vi "Subtract DAQ Offset.vi"(8 "error in (no error)":errorcluster, 11 "Instrument.DAQ":refnum<class "Instrument.DAQ.lvclass">) -> (0 "error out":errorcluster, 3 "Instrument.DAQ out":refnum<class "Instrument.DAQ.lvclass">)   [LabVIEW 2019, in "Instrument.Lockin.lvlib" / "Instrument.DAQ.lvclass"]
uses:
  Instrument.DAQ.lvclass
  Instrument.DAQ.lvclass/Instrument.DAQ.ctl
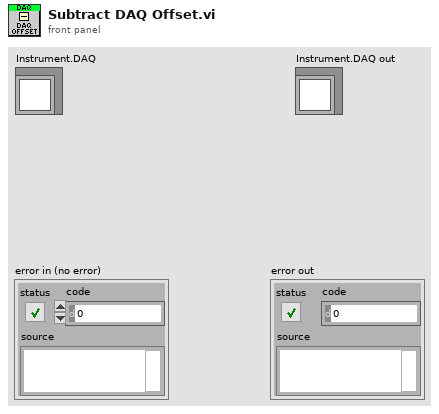
[diagram p1: front panel]
types:
  T1 = typedef "Instrument.Lockin.lvlib/Instrument.DAQ.lvclass/Channel.Gain--Cluster--Array.ctl" = T2[]
  T2 = typedef "Instrument.Lockin.lvlib/Instrument.DAQ.lvclass/Channel.Gain--Cluster.ctl" = cluster{"Channel":string, "Gain":dbl}
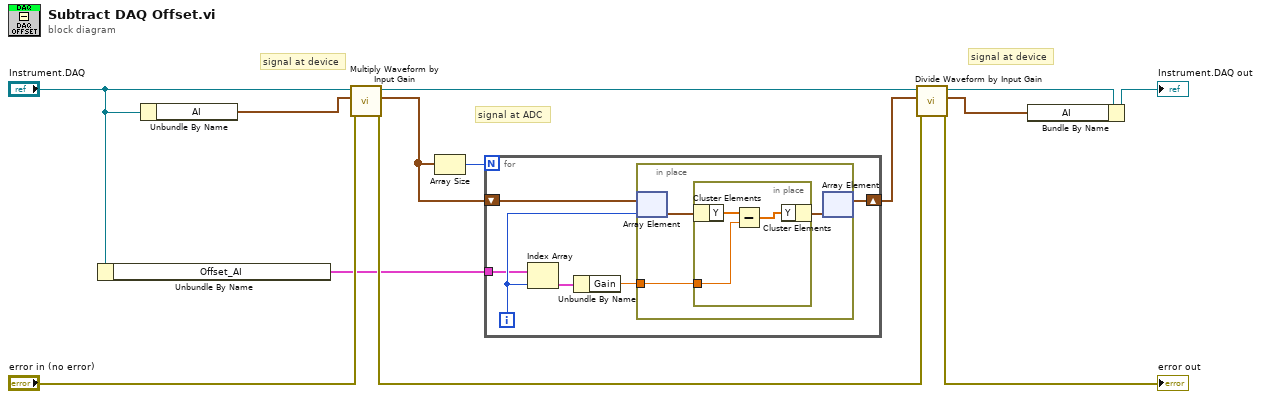
[diagram p0: block diagram]
diagram:
  # "signal at device"
  # "signal at ADC"
  # "signal at device"
  n1 = Unbundle By Name("Instrument.DAQ") -> ("Offset_AI"=w6:T1)
  n2 = Unbundle By Name("Instrument.DAQ") -> ("AI"=w4:waveform(dbl)[])
  n3 = call "Multiply Waveform by Input Gain.vi"("error in (no error)"="error in (no error)", "WFM in"=w4, "Instrument.DAQ"="Instrument.DAQ") -> ("error out"=w8:errorcluster, "WFM out"=w7:waveform(dbl)[], "Instrument.DAQ out"=w3:refnum<class "Instrument.DAQ.lvclass">)  [unwired: 6 in]
  n4 = Array Size(array=w7) -> (size(s)=w10:i32)
  n5 = for {
    N: w10 -> [_]
    tunnel: w6 -> [w16]
    shift-right: [w18] -> w9
    shift-left: w7 -> [w19]
    i -> [w17]
    n6 = Index Array(array=w16, index=w17) -> (element=w15:T2)
    n7 = Unbundle By Name(w15) -> ("Gain"=w14:dbl)
    n8 = in-place {
      in-place-border: w14 -> [w22]
      n9 = in-place-array #1(w19, w17) -> (w21:waveform(dbl))
      n10 = in-place {
        in-place-border: w22 -> [w23]
        n11 = in-place-cluster #2(w21) -> ("Y"=w25:dbl[])
        n12 = Subtract(x=w25, y=w23) -> (x-y=w24:dbl[])
        n13 = in-place-cluster #2("Y"=w24) -> (w20:waveform(dbl))
      }
      n14 = in-place-array #1(w20) -> (w18:waveform(dbl)[])  [unwired: 1 out]
    }
  }
  n15 = call "Divide Waveform by Input Gain.vi"("error in (no error)"=w8, "WFM in"=w9, "Instrument.DAQ"=w3) -> ("error out"=→"error out":errorcluster, "WFM out"=w5:waveform(dbl)[], "Instrument.DAQ out"=w2:refnum<class "Instrument.DAQ.lvclass">)  [unwired: 6 in]
  n16 = Bundle By Name(cluster=w2, "AI"=w5) -> (→"Instrument.DAQ out":refnum<class "Instrument.DAQ.lvclass">)
